vi "FPGA.vi"() -> ()   [LabVIEW 2015]
uses:
  <vilib>/EmbeddedDisplay/Hitachi HD44780/Common/Control/lcd command cluster.ctl
  <vilib>/EmbeddedDisplay/Hitachi HD44780/Common/Control/8bit connection map.ctl
  <vilib>/rvi/Emulation/niFpgaGetClockAttributes.vi
  <vilib>/rvi/Emulation/niFpgaSctlEmulationGetInTimedLoop.vi
  <vilib>/rvi/Emulation/niFpgaEmulationReportErrorSimple.vi
  <vilib>/EmbeddedDisplay/Hitachi HD44780/FPGA/Internal/LCD Command.vi
  <vilib>/EmbeddedDisplay/Hitachi HD44780/FPGA/Public/Command Handler (8 Bits).vi
  <vilib>/rvi/Emulation/niFpgaProcessEmulError.vi
  <vilib>/rvi/Emulation/niFpgaCriticalErrorInLSC.vi
  <vilib>/EmbeddedDisplay/Hitachi HD44780/Common/HD44780 Common.lvlib
  <vilib>/EmbeddedDisplay/Hitachi HD44780/FPGA/HD44780 FPGA.lvlib
panel:
  in  "LCD Command":T1={"device index (-1)"=-1, "operation (0)"=0}
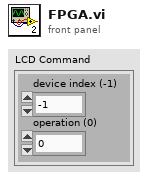
[diagram p1: front panel]
types:
  T1 = typedef "HD44780 Common.lvlib/lcd command cluster.ctl" = cluster{"device index (-1)":i8, "operation (0)":u32}
  T2 = typedef "HD44780 Common.lvlib/8bit connection map.ctl" = cluster{"RS":refnum<k21>, "R/W":refnum<k21>, "E1":refnum<k21>, "E2":refnum<k21>, "DB0":refnum<k21>, "DB1":refnum<k21>, "DB2":refnum<k21>, "DB3":refnum<k21>, "DB4":refnum<k21>, "DB5":refnum<k21>, "DB6":refnum<k21>, "DB7":refnum<k21>}
  T3 = cluster{"device index (-1)":i8, "operation (0)":u32}
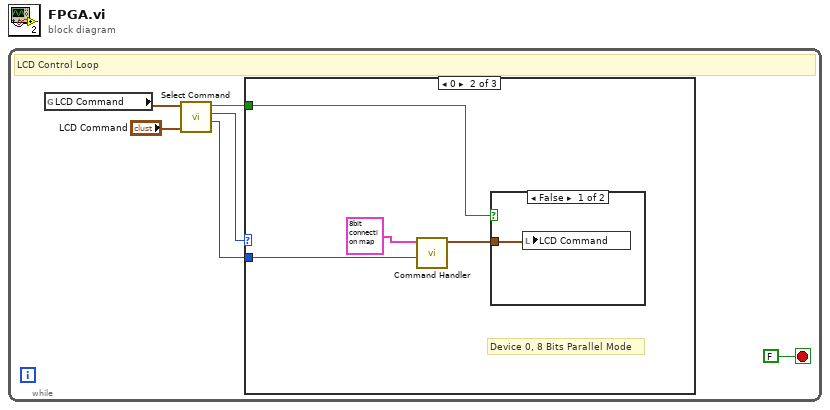
[diagram p0: block diagram]
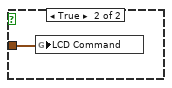
[diagram p3: hidden frame]
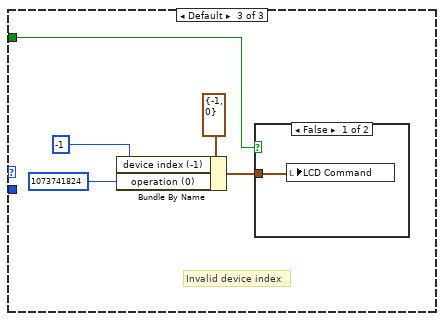
[diagram p4: hidden frame]
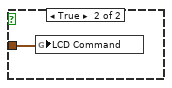
[diagram p5: hidden frame]
diagram:
  n1 = while {
    stop <- FALSE stop-if-true
    # "LCD Control Loop"
    n2 = global read "LCD Command.vi" "LCD Command"() -> (w2:T3)
    n3 = call <vilib>:"Select Command.vi"("Host LCD Command"="LCD Command", "FPGA LCD Command"=w2) -> ("operation"=w4:u32, "device index"=w5:i8, "FPGA? True : False"=w3:bool)  [unwired: 7 in]
    n4 = case shown="0" w5 {
      tunnel: w4 -> [_ w10 _]
      tunnel: w3 -> [_ w9 w17]
      frame -1 {
        # "IDLE State"
      }
      frame 0 {
        # "Device 0, 8 Bits Parallel Mode"
        n5 = call-poly <vilib>:"Command Handler.vi"("operation"=w10, "device connection map in"=T2 {"RS"="DIO19", "R/W"="DIO18", "E1"="DIO17", "E2"="DIO17", "DB0"="DIO20", "DB1"="DIO21", "DB2"="DIO22", "DB3"="DIO23", "DB4"="DIO24", "DB5"="DIO25", "DB6"="DIO26", "DB7"="DIO27"}) -> ("result"=w8:T3)  [unwired: 9 in]
        n6 = case shown="False" w9 {
          tunnel: w8 -> [w11 w12]
          frame False {
            n7 = local write "LCD Command"(w11) -> ()
          }
          frame True {
            n8 = global write "LCD Command.vi" "LCD Command"(w12) -> ()
          }
        }
      }
      frame Default {
        # "Invalid device index"
        n9 = Bundle By Name(cluster=T1 {"device index (-1)"=-1, "operation (0)"=0} ("LCD Command"), "device index (-1)"=i8 -1 ("LCD_device index (-1)"), "operation (0)"=u32 1073741824 ("LCD_operation (0)")) -> (w13:T1)
        n10 = case shown="False" w17 {
          tunnel: w13 -> [w18 w19]
          frame False {
            n11 = local write "LCD Command"(w18) -> ()
          }
          frame True {
            n12 = global write "LCD Command.vi" "LCD Command"(w19) -> ()
          }
        }
      }
    }
  }
